vi "S2C_FORNAX_Poly_SupervisorCommand.vi"(8 "Error In":errorcluster, 10 "SupervisorCommand":T1={"Partition"="Default", "Message"="SupervisorCommand", "M_ModuleId"=0, "M_SupervisorCommandAction"=0, "M_SequenceId"=0}, 11 "Settings":T2={"Driver"="Fornax", "Command"="SupervisorCommand", "Return"="ErrorStatus", "Parameters"="", "Timeout"=10.0}) -> (0 "Error Out":errorcluster, 3 "Response":string)   [LabVIEW 2015]
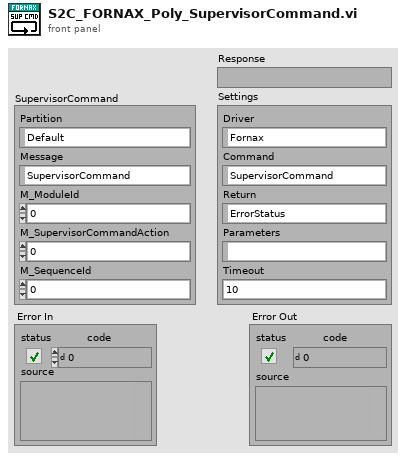
[diagram p1: front panel]
types:
  T1 = cluster{"Partition":string, "Message":string, "M_ModuleId":i32, "M_SupervisorCommandAction":i32, "M_SequenceId":i32}
  T2 = cluster{"Driver":string, "Command":string, "Return":string, "Parameters":string, "Timeout":dbl}
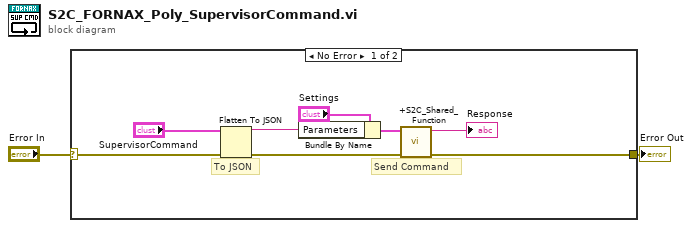
[diagram p0: block diagram]
diagram:
  n1 = case shown="No Error" "Error In" {
    selector: "Error In" -> [w6 w11]
    tunnel: [w5 w11] -> w1
    frame No Error {
      # "To JSON"
      # "Send Command"
      n2 = Flatten To JSON(anything="SupervisorCommand", error in (no error)=w6) -> (JSON string=w7:string, 11:w9:errorcluster)  [unwired: 1 in]
      n3 = Bundle By Name(cluster="Settings", "Parameters"=w7) -> (w10:T2)
      n4 = call "+S2C_Shared_Function.vi"("Error In"=w9, "Settings"=w10) -> ("Error Out"=w5:errorcluster, "Response"=→"Response":string)  [unwired: 8 in]
    }
    frame Error {
    }
  }
  "Error Out" <- w1
